vi "GetPictureData.vi"(5 "Resolution":cluster{"Width":u32, "Height":u32}, 6 "Data(8Bit)":u8[](array[numeric]), 7 "ColorType":enum16{"MONO", "COLOR"}(ring)) -> (3 "new picture":picture)   [LabVIEW 2015]
uses:
  <vilib>/picture/picture.llb/imagedata.ctl
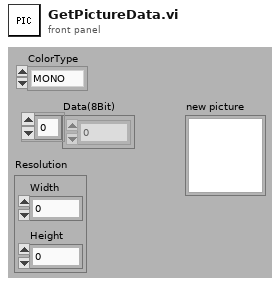
[diagram p1: front panel]
types:
  T1 = typedef "imagedata.ctl" = cluster{"image type":i32, "image depth":i32, "image":u8[], "mask":u8[], "colors":u32[], "Rectangle":cluster{"left":i16, "top":i16, "right":i16, "bottom":i16}}
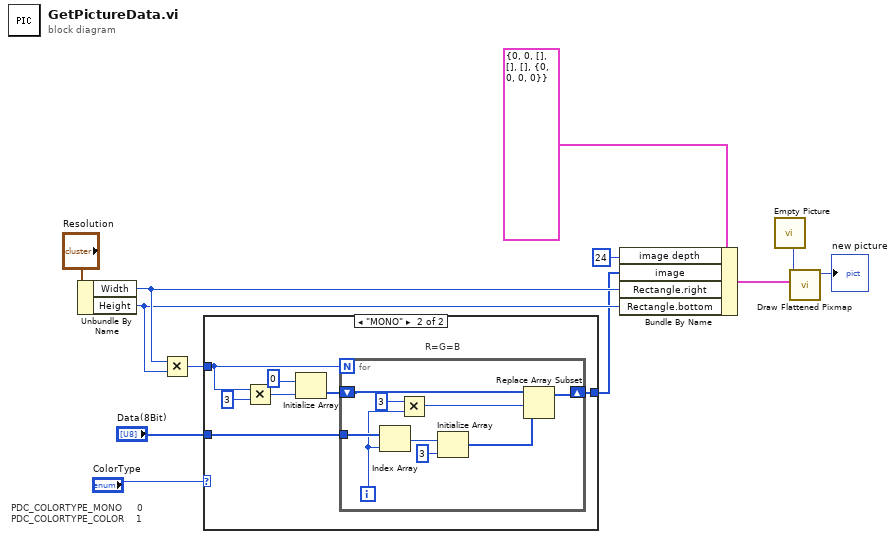
[diagram p0: block diagram]
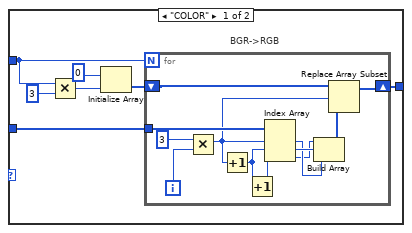
[diagram p2: hidden frame]
diagram:
  # "PDC_COLORTYPE_MONO\t\t\t\t\t0\nPDC_COLORTYPE_COLOR\t\t\t\t1"
  n1 = Unbundle By Name("Resolution") -> ("Width"=w8:u32, "Height"=w7:u32)
  n2 = Multiply(x=w8, y=w7) -> (x*y=w9:u32)
  n3 = case shown="\"MONO\"" "ColorType" {
    tunnel: w9 -> [w18 w37]
    tunnel: [w14 w33] -> w6
    tunnel: "Data(8Bit)" -> [w13 w32]
    frame "COLOR" {
      # "BGR->RGB"
      n4 = Multiply(x=w18, y=3) -> (x*y=w16:u32)
      n5 = Initialize Array(u8 0, w16) -> (w15:u8[])
      n6 = for {
        N: w18 -> [_]
        shift-right: [w22] -> w14
        shift-left: w15 -> [w23]
        tunnel: w13 -> [w31]
        i -> [w26]
        n7 = Multiply(x=3, y=w26) -> (x*y=w20:i32)
        n8 = Increment(x=w20) -> (x+1=w25:i32)
        n9 = Increment(x=w25) -> (x+1=w24:i32)
        n10 = Index Array(array=w31, index #1=w20, index #2=w25, index #3=w24) -> (element #1=w29:u8, element #2=w30:u8, element #3=w28:u8)
        n11 = Build Array(w28, w30, w29) -> (w21:u8[])
        n12 = Replace Array Subset(array=w23, new element=w21, index=w20) -> (w22:u8[])
      }
    }
    frame "MONO" {
      # "R=G=B"
      n13 = Multiply(x=w37, y=3) -> (x*y=w35:u32)
      n14 = Initialize Array(u8 0, w35) -> (w34:u8[])
      n15 = for {
        N: w37 -> [_]
        shift-right: [w44] -> w33
        shift-left: w34 -> [w45]
        tunnel: w32 -> [w47]
        i -> [w42]
        n16 = Index Array(array=w47, index=w42) -> (element=w41:u8)
        n17 = Multiply(x=3, y=w42) -> (x*y=w43:i32)
        n18 = Initialize Array(w41, 3 ("次元サイズ")) -> (w39:u8[])
        n19 = Replace Array Subset(array=w45, new element=w39, index=w43) -> (w44:u8[])
      }
    }
  }
  n20 = Bundle By Name(cluster=T1 {"image type"=0, "image depth"=0, "image"=[], "mask"=[], "colors"=[], "Rectangle"={"left"=0, "top"=0, "right"=0, "bottom"=0}} ("image data"), "image depth"=24, "image"=w6, "Rectangle.right"=w8, "Rectangle.bottom"=w7) -> (w12:T1)
  n21 = call "Empty Picture"() -> ("empty picture"=w1:picture)
  n22 = call <vilib>:"Draw Flattened Pixmap.vi"("image data"=w12, "picture"=w1) -> ("new picture"=→"new picture":picture)  [unwired: 7 out]
